vi "PS35_MotorCommCounts.vi"(0 "Axis number":i32=1 min=1 max=3, 1 "Control unit ID":i32=1 min=1 max=10, 2 "Value-In":i32=1 min=1 max=65535, 3 "error in (no error)":errorcluster, 5 "function":bool) -> (7 "Value-Out":i32, 9 "error out":errorcluster)   [LabVIEW 2020]
doc: "PS35_MotorCommCounts.vi, created: 04.03.2009 alex; last change: 22.10.2019 alex;\n\n<B>FUNCTIONS:</B> \n\n<B>Read:</B> FALSE: read encoder counts of an axis \nfor a commutating cycle.\n<B>Write:</B> TRUE: set encoder counts of an axis\nfor a commutating cycle.\nThis is valid only for the step motor axes (Closed-Loop).\n----------------------------------------------------------------------------------------\n<B>INPUT:</B>\n[TF] <B>function:</B> function selector. (Read, Write)\n[I32] <B>Control unit ID:</B> control unit index. (Default=1, Range=1...10)\n[I32] <B>Axis number:</B> axis number. (Default=1, Range=1...3)\n[I32] <B>Value-In:</B> encoder counts. \n(only for Write: Default=1, Range=1...65535)\n[CLU] <B>error in</B>\n----------------------------------------------------------------------------------------\n<B>OUTPUT:</B>\n[I32] <B>Value-Out:</B> encoder counts. (for Write: Value-Out=Value-In)\n[CLU] <B>error out</B>\n----------------------------------------------------------------------------------------\n<B>SUB-VIs:</B>\nPS35_GetReadError.vi\n----------------------------------------------------------------------------------------\n<B>EXT-Calls:</B>\nps35.dll (V2.01)\n----------------------------------------------------------------------------------------"
uses:
  ps35.dll
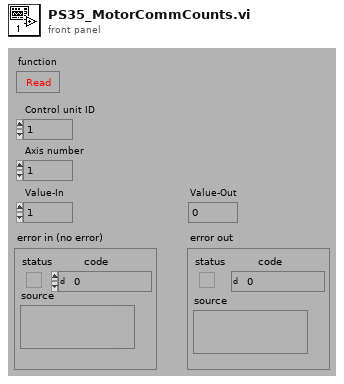
[diagram p1: front panel]
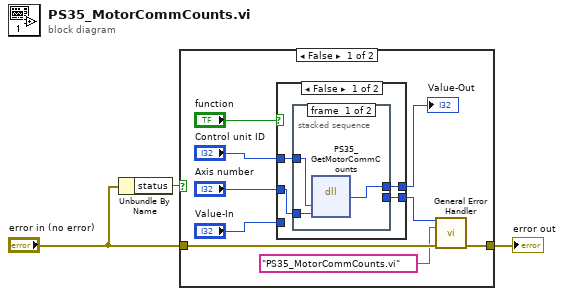
[diagram p0: block diagram]
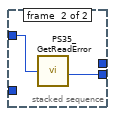
[diagram p2: hidden frame]
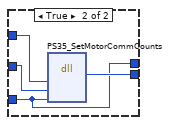
[diagram p3: hidden frame]
diagram:
  n1 = Unbundle By Name("error in (no error)") -> ("status"=w1:bool)
  n2 = case shown="False" w1 {
    tunnel: "error in (no error)" -> [w12 w26]
    tunnel: [w11 w26] -> w3
    frame False {
      n3 = case shown="False" "function" {
        tunnel: "Control unit ID" -> [w15 w24]
        tunnel: [w16 w25] -> w8
        tunnel: "Value-In" -> [_ w22]
        tunnel: [w14 w22] -> w6
        tunnel: "Axis number" -> [w13 w23]
        frame False {
          n4 = stacked-sequence {
            tunnel: [_ w21] -> w16
            tunnel: w15 -> [w19 w20]
            tunnel: [w18 _] -> w14
            tunnel: w13 -> [w17 _]
            frame #0 {
              n5 = dll-call lib="C:/GEECS/Developers Version/source/Device Drivers/OwiSoft/OWISoftOEM/ps35/labview/lv82/ps35.dll" fn="PS35_GetMotorCommCounts" label="PS35_Get\nMotorComm\nCounts"("Index"=w19, "AxisNr"=w17) -> ("Rückgabetyp"=w18:i32)  [unwired: 5 in, 2 out]
            }
            frame #1 {
              n6 = call "PS35_GetReadError.vi"("Control unit ID"=w20) -> ("Read error"=w21:i32)
            }
          }
        }
        frame True {
          n7 = dll-call lib="C:/GEECS/Developers Version/source/Device Drivers/OwiSoft/OWISoftOEM/ps35/labview/lv82/ps35.dll" fn="PS35_SetMotorCommCounts" label="PS35_Set\nMotorComm\nCounts"("Index"=w24, "AxisNr"=w23, "Value"=w22) -> ("Rückgabetyp"=w25:i32)  [unwired: 6 in, 2 out]
        }
      }
      "Value-Out" <- w6
      n8 = call <vilib>:"General Error Handler.vi"("[error code] (0)"=w8, "[error source] (\" \")"="PS35_MotorCommCounts.vi" ("[error source] (\" \")"), "error in (no error)"=w12) -> ("error out"=w11:errorcluster)  [unwired: 8 in, 4 out]
    }
    frame True {
    }
  }
  "error out" <- w3
